vi "clog.vi"(4 "error":errorcluster) -> ()   [LabVIEW 2010]
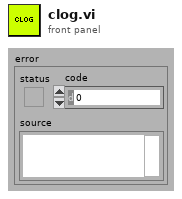
[diagram p1: front panel]
types:
  T1 = cluster{"seconds since 1Jan1904":timestamp, "error IO":errorcluster}
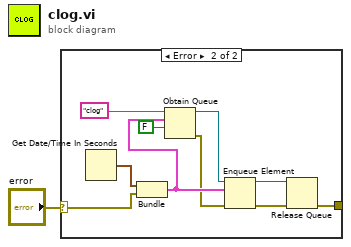
[diagram p0: block diagram]
diagram:
  n1 = case shown="Error" "error" {
    selector: "error" -> [_ w10]
    tunnel: [_ w4] -> _
    frame No Error {
    }
    frame Error {
      n2 = Get Date/Time In Seconds() -> (seconds since 1Jan1904=w11:timestamp)
      n3 = Bundle("seconds since 1Jan1904"=w11, "error IO"=w10) -> (w8:T1)  [unwired: 1 in]
      n4 = Obtain Queue(name (unnamed)="clog", element data type=w8, create if not found? (T)=FALSE) -> (queue out=w7:refnum<queue>, error out=w6:errorcluster)  [unwired: 2 in, 1 out]
      n5 = Enqueue Element(queue=w7, element=w8, error in (no error)=w6) -> (queue out=w3:refnum<queue>, error out=w5:errorcluster)  [unwired: 1 in, 1 out]
      n6 = Release Queue(queue=w3, error in (no error)=w5) -> (error out=w4:errorcluster)  [unwired: 1 in, 2 out]
    }
  }
